vi "Bob Action.vi"(8 "error in (no error)":errorcluster, 11 "Bob in":refnum<class "Bob.lvclass">) -> (0 "error out":errorcluster, 3 "Bob out":refnum<class "Bob.lvclass">)   [LabVIEW 2014, in "Bob.lvlib" / "Bob.lvclass"]
uses:
  Bob.lvclass
panel:
  # "Bob Action"
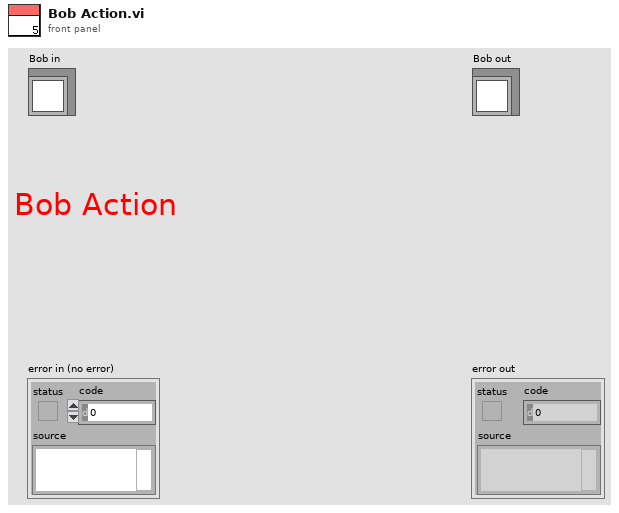
[diagram p1: front panel]
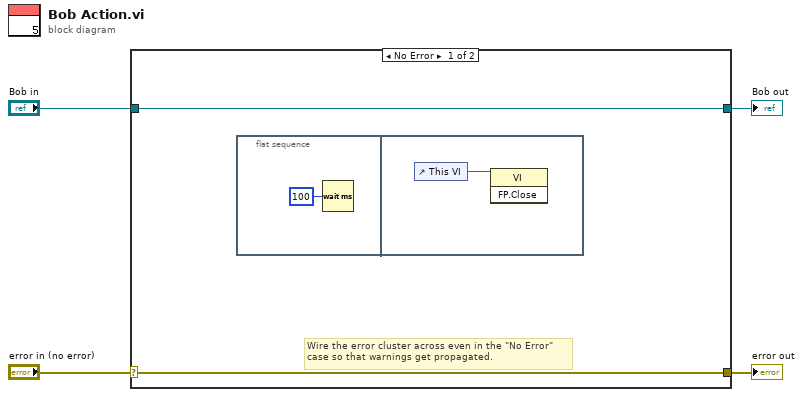
[diagram p0: block diagram]
diagram:
  n1 = case shown="No Error" "error in (no error)" {
    selector: "error in (no error)" -> [w5 w10]
    tunnel: [w5 w10] -> w3
    tunnel: [w6 w9] -> w1
    tunnel: "Bob in" -> [w6 w9]
    frame No Error {
      # "Wire the error cluster across even in the \"No Error\"\ncase so that warnings get propagated."
      n2 = flat-sequence {
        frame #0 {
          n3 = Wait (ms)(milliseconds to wait=u32 100) -> ()  [unwired: 1 out]
        }
        frame #1 {
          n4 = control-ref of="This VI"() -> (w8:refnum<vi>)
          n5 = invoke class="VI" method="FP.Close"(reference=w8) -> ()  [unwired: 2 in, 3 out]
        }
      }
    }
    frame Error {
    }
  }
  "error out" <- w3
  "Bob out" <- w1
